vi "AlazarNumOfSystems.vi"(0 "error in (no error)":errorcluster) -> (1 "System Count":u32, 2 "error out":errorcluster)   [LabVIEW 2009]
doc: "Get the total number of board systems detected."
uses:
  ATSApi.dll
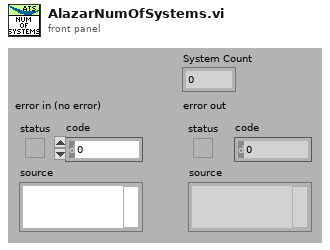
[diagram p1: front panel]
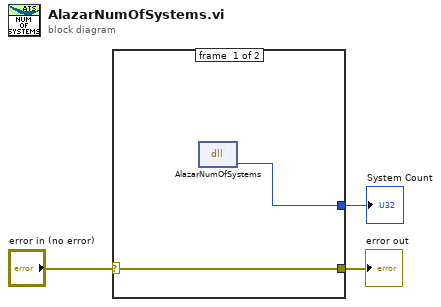
[diagram p0: block diagram]
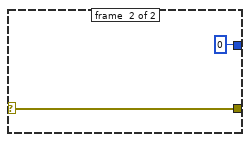
[diagram p2: hidden frame]
diagram:
  n1 = case shown="No Error" "error in (no error)" {
    selector: "error in (no error)" -> [w4 w7]
    tunnel: [w4 w7] -> w2
    tunnel: [w5 u32 0] -> w1
    frame #0 {
      n2 = dll-call lib="ATSApi.dll" fn="AlazarNumOfSystems"() -> (w5:u32)  [unwired: 3 in, 2 out]
    }
    frame #1 {
    }
  }
  "error out" <- w2
  "System Count" <- w1
